vi "InsightTelnetOpenClose.vi"(0 "telnet connection":T1, 1 "IP Address":string="192.168.0.222", 2 "remote port (23)":u16=23, 3 "error in (no error)":errorcluster, 4 "Method":enum16{"Telnet Open", "Telnet Close"}(ring), 6 "line separator":string="atlas ready>") -> (7 "telnet connection":T1, 10 "error out":errorcluster)   [LabVIEW 2014]
doc: "This VI opens or closes telnet communications to the Insight laser."
uses:
  Telnet Session.ctl
panel:
  out "data out":string
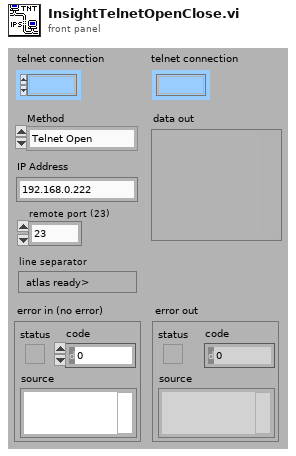
[diagram p1: front panel]
types:
  T1 = typedef "Telnet Session.ctl" = refnum<k1>
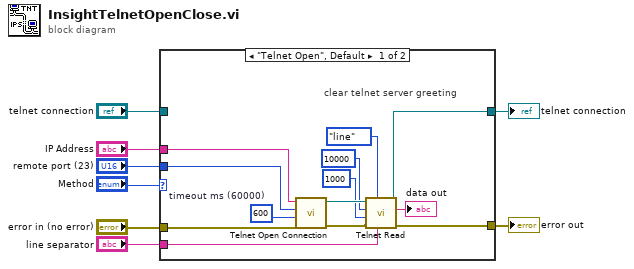
[diagram p0: block diagram]
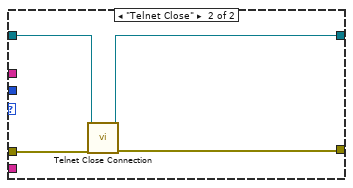
[diagram p2: hidden frame]
diagram:
  n1 = case shown="\"Telnet Open\", Default" "Method" {
    tunnel: "error in (no error)" -> [w21 w25]
    tunnel: "IP Address" -> [w20 _]
    tunnel: [w17 w24] -> w5
    tunnel: "telnet connection" -> [_ w23]
    tunnel: [w15 w22] -> w3
    tunnel: "line separator" -> [w11 _]
    tunnel: "remote port (23)" -> [w9 _]
    frame "Telnet Open", Default {
      w19 = 600  # timeout ms (60000)
      # "clear telnet server greeting"
      n2 = call "Telnet Open Connection.vi"("error in (no error)"=w21, "timeout ms (60000)"=w19, "remote port (23)"=w9, "address"=w20) -> ("error out"=w18:errorcluster, "telnet connection"=w16:T1)  [unwired: 6 in]
      n3 = call "Telnet Read.vi"("line separator"=w11, "read mode (normal)"=enum16{"normal", "line", "buffered"}."line", "error in (no error)"=w18, "timeout ms (25000)"=1000, "bytes to read"=10000, "telnet connection"=w16) -> ("error out"=w17:errorcluster, "data out"=→"data out":string, "telnet connection out"=w15:T1)  [unwired: 1 in]
    }
    frame "Telnet Close" {
      n4 = call "Telnet Close Connection.vi"("error in (no error)"=w25, "telnet connection"=w23) -> ("error out"=w24:errorcluster, "telnet connection out"=w22:T1)  [unwired: 8 in]
    }
  }
  "error out" <- w5
  "telnet connection" <- w3
